vi "HP34401_get_4wR.vi"(8 "error in":errorcluster, 10 "timeout [ms]":i32=5000, 11 "VISA in":refnum<visa-resource-name>) -> (0 "error out":errorcluster, 2 "Measurement":dbl, 3 "VISA out":refnum<visa-resource-name>)   [LabVIEW 2020]
uses:
  drivers/HP34401A/Public/Data/Read (Single Point).vi
  drivers/HP34401A/Agilent 34401.lvlib
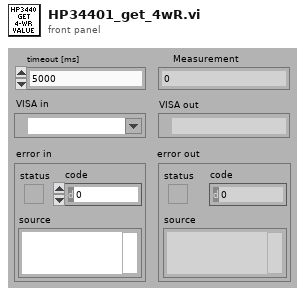
[diagram p1: front panel]
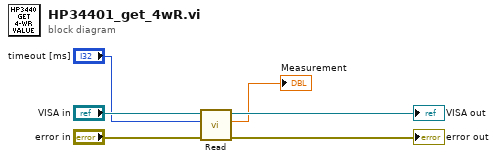
[diagram p0: block diagram]
diagram:
  n1 = call-poly "Read.vi"("error in (no error)"="error in", "timeout [ms]"="timeout [ms]", "VISA resource name"="VISA in") -> ("error out"=→"error out":errorcluster, "Measurement"=→"Measurement":dbl, "VISA resource name out"=→"VISA out":refnum<visa-resource-name>)  [unwired: 6 in]
